vi "DialCreate.vi"(11 "Solid Horizon Path.PNG":path=path "C:/Users/uksayerr/Documents/My LabView/Content Creation/artificial horizon/FixedHorizonTrans.png") -> (3 "SceneObject out":refnum<vi>)   [LabVIEW 2015]
uses:
  <vilib>/picture/3D Picture Control/Object/Create Object (name).vi
  <vilib>/picture/3D Picture Control/NI_3D Picture Control.lvlib
panel:
  # "Generates the Dial with the picture \nat the path specified below"
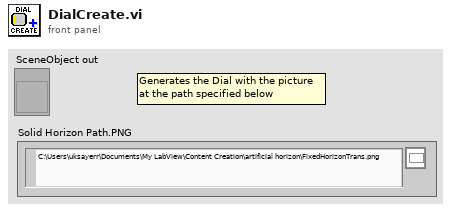
[diagram p1: front panel]
types:
  T1 = enum16{"As a Decal", "With Modulation", "With Blending", "As a replacement"}
  T2 = cluster{"Red":sgl, "Green":sgl, "Blue":sgl, "Alpha":sgl}[]
  T3 = enum16{"Overall", "Per Primitive", "Per Vertex", "Binding Off"}
  T4 = enum16{"Normal Bin", "Opaque Bin", "Transparent Bin"}
  T5 = enum16{"Points", "Lines", "Line Strip", "Line Loop", "Triangles", "Triangle Strip", "Triangle Fan", "Quads", "Quad Strip", "Polygon"}
  T6 = typedef "imagedata.ctl" = cluster{"image type":i32, "image depth":i32, "image":u8[], "mask":u8[], "colors":u32[], "Rectangle":cluster{"left":i16, "top":i16, "right":i16, "bottom":i16}}
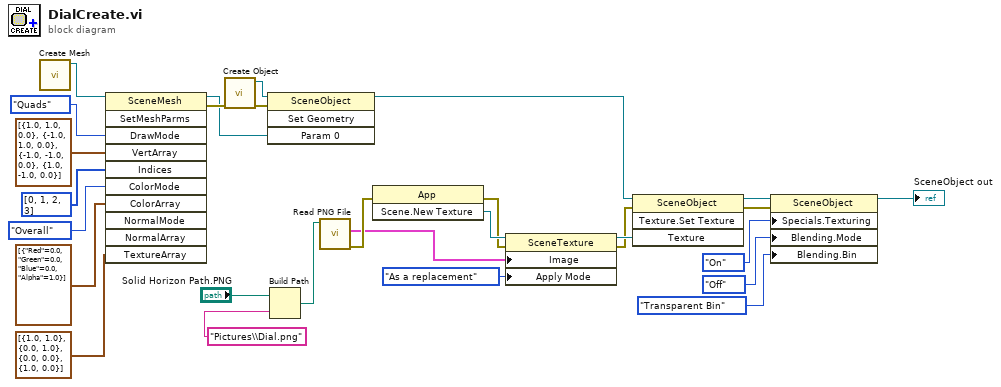
[diagram p0: block diagram]
diagram:
  n1 = call <vilib>:"Create Mesh.vi"() -> ("New Mesh Refnum"=w18:refnum<vi>)  [unwired: 10 in, 1 out]
  n2 = invoke class="SceneMesh" method="SetMeshParms"(reference=w18, "DrawMode"=T5."Quads" ("Draw Mode"), "VertArray"=cluster{"X":sgl, "Y":sgl, "Z":sgl}[] [{"X"=1.0, "Y"=1.0, "Z"=0.0}, {"X"=-1.0, "Y"=1.0, "Z"=0.0}, {"X"=-1.0, "Y"=-1.0, "Z"=0.0}, {"X"=1.0, "Y"=-1.0, "Z"=0.0}] ("Vertex Array"), "Indices"=u32[] [0, 1, 2, 3], "ColorMode"=T3."Overall" ("Color Binding Mode"), "ColorArray"=T2 [{"Red"=0.0, "Green"=0.0, "Blue"=0.0, "Alpha"=1.0}] ("Color Array"), "TextureArray"=cluster{"S":sgl, "T":sgl}[] [{"S"=1.0, "T"=1.0}, {"S"=0.0, "T"=1.0}, {"S"=0.0, "T"=0.0}, {"S"=1.0, "T"=0.0}] ("Texture Coordinate Array")) -> (reference out=w12:refnum<vi>, error out=w14:errorcluster)  [unwired: 4 in, 9 out]
  n3 = call-poly <vilib>:"Create Object.vi"("error in (no error)"=w14) -> ("error out"=w13:errorcluster, "Scene:New Object"=w25:refnum<vi>)  [unwired: 9 in]
  n4 = invoke class="SceneObject" method="Set Geometry"(reference=w25, error in=w13, "Param 0"=w12) -> (reference out=w24:refnum<vi>)  [unwired: 1 in, 3 out]
  n5 = Build Path(base path="Solid Horizon Path.PNG", name or relative path="Pictures\\Dial.png") -> (appended path=w1:path)
  n6 = call <vilib>:"Read PNG File.vi"("path to PNG file"=w1) -> ("error out"=w20:errorcluster, "image data"=w19:T6)  [unwired: 8 in, 1 out]
  n7 = invoke class="App" method="Scene.New Texture"(error in=w20) -> (error out=w22:errorcluster, "Scene.New Texture"=w23:refnum<vi>)  [unwired: 2 in, 1 out]
  n8 = property class="SceneTexture"(reference=w23, error in=w22, "Image"=w19, "Apply Mode"=T1."As a replacement") -> (reference out=w11:refnum<vi>, error out=w10:errorcluster)
  n9 = invoke class="SceneObject" method="Texture.Set Texture"(reference=w24, error in=w10, "Texture"=w11) -> (reference out=w9:refnum<vi>, error out=w8:errorcluster)  [unwired: 1 in, 2 out]
  n10 = property class="SceneObject"(reference=w9, error in=w8, "Specials.Texturing"=enum16{"Inherit Value", "Off", "On"}."On" ("Specials:Texturing"), "Blending.Mode"=enum16{"Inherit Value", "Off", "On"}."Off" ("Blending:Mode 2"), "Blending.Bin"=T4."Transparent Bin" ("Blending:Bin")) -> (reference out=→"SceneObject out":refnum<vi>)  [unwired: 1 out]
